vi "To Pretty String (Array).vi"(6 "pretty print? (T)":bool=TRUE, 7 "enable LabVIEW extensions? (T)":bool=TRUE, 8 "error in (no error)":errorcluster, 10 "indent":i32, 11 "JSON Value in":refnum<class "JSON Value.lvclass">) -> (0 "error out":errorcluster, 3 "Pretty Print String":string)   [LabVIEW 2016, in "JSON Value.lvclass"]
doc: "Pretty prints the given JSON data in an easier to read format."
uses:
  JSON Value.lvclass
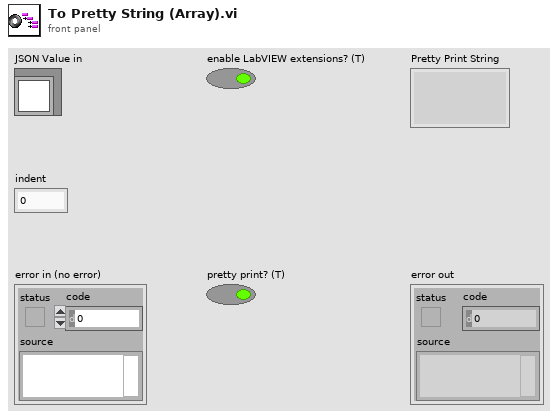
[diagram p1: front panel]
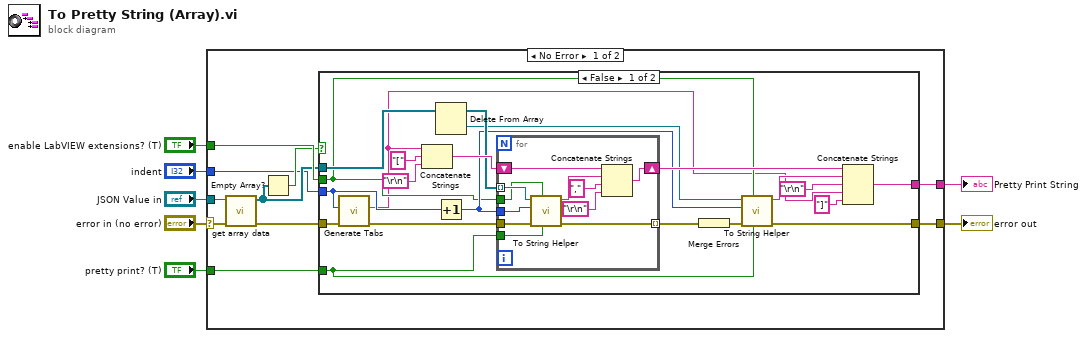
[diagram p0: block diagram]
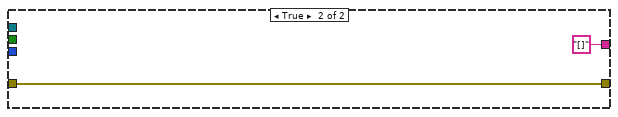
[diagram p2: hidden frame]
diagram:
  n1 = case shown="No Error" "error in (no error)" {
    selector: "error in (no error)" -> [w13 w52]
    tunnel: [w17 _] -> w7
    tunnel: [w16 w52] -> w6
    tunnel: "enable LabVIEW extensions? (T)" -> [w15 _]
    tunnel: "JSON Value in" -> [w14 _]
    tunnel: "indent" -> [w9 _]
    tunnel: "pretty print? (T)" -> [w8 _]
    frame No Error {
      n2 = call "get array data.vi"("error in (no error)"=w13, "JSON Value in"=w14) -> ("error out"=w12:errorcluster, "JSON Array out"=w10:refnum<class "JSON Value.lvclass">[])  [unwired: 8 in]
      n3 = Empty Array?(array=w10) -> (empty?=w11:bool)
      n4 = case shown="False" w11 {
        tunnel: [w38 "[]"] -> w17
        tunnel: [w23 w50] -> w16
        tunnel: w10 -> [w28 _]
        tunnel: w15 -> [w21 _]
        tunnel: w12 -> [w37 w50]
        tunnel: w9 -> [w36 _]
        tunnel: w8 -> [w22 _]
        frame False {
          n5 = call "Generate Tabs.vi"("error in (no error)"=w37, "indent"=w36) -> ("error out"=w34:errorcluster, "Tabs"=w18:string)  [unwired: 8 in]
          n6 = Concatenate Strings(w18, "[" ("string"), "\r\n") -> (w32:string)
          n7 = Delete From Array(array=w28) -> (deleted portion=w26:refnum<class "JSON Value.lvclass">, array with subset deleted=w27:refnum<class "JSON Value.lvclass">[])  [unwired: 2 in]
          n8 = Increment(x=w36) -> (x+1=w25:i32)
          n9 = for {
            tunnel: w27 -> [w49] mode=indexing
            tunnel: w25 -> [w48]
            tunnel: w34 -> [w47]
            shift-right: [w45] -> w31
            shift-left: w32 -> [w44]
            tunnel: [w43] -> w30 mode=indexing
            tunnel: w22 -> [w42]
            tunnel: w21 -> [w41]
            n10 = call "To String Helper.vi"("pretty print? (T)"=w42, "enable LabVIEW extensions? (T)"=w41, "error in (no error)"=w47, "indent"=w48, "JSON Value in"=w49) -> ("error out"=w43:errorcluster, "String"=w46:string)  [unwired: 5 in]
            n11 = Concatenate Strings(w44, w46, "," ("string"), "\r\n") -> (w45:string)
          }
          n12 = Merge Errors(w30) -> (w24:errorcluster)
          n13 = call "To String Helper.vi"("pretty print? (T)"=w22, "enable LabVIEW extensions? (T)"=w21, "error in (no error)"=w24, "indent"=w25, "JSON Value in"=w26) -> ("error out"=w23:errorcluster, "String"=w20:string)  [unwired: 5 in]
          n14 = Concatenate Strings(w31, w20, "\r\n", w18, "]" ("string")) -> (w38:string)
        }
        frame True {
        }
      }
    }
    frame Error {
    }
  }
  "error out" <- w6
  "Pretty Print String" <- w7
